vi "Take Your Seat.vi"(8 "error in (no error)":errorcluster, 10 "Front Panel Window:Panel Bounds":T1, 11 "Philosopher in":refnum<class "Philosopher.lvclass">) -> (0 "error out":errorcluster, 3 "Philosopher out":refnum<class "Philosopher.lvclass">)   [LabVIEW 2023, in "Philosopher.lvlib" / "Philosopher.lvclass"]
uses:
  Philosopher.lvclass
  <vilib>/Utility/miscctls.llb/LVRectTypeDef.ctl
  Philosopher.lvclass/Philosopher.ctl
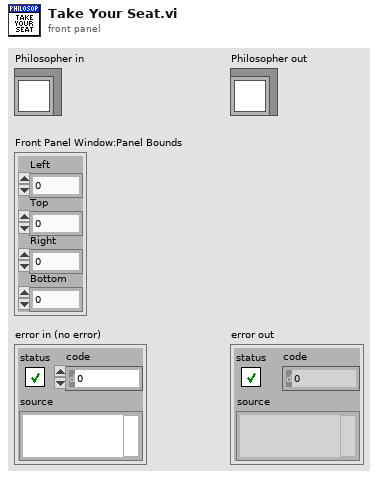
[diagram p1: front panel]
types:
  T1 = typedef "LVRectTypeDef.ctl" = cluster{"Left":i16, "Top":i16, "Right":i16, "Bottom":i16}
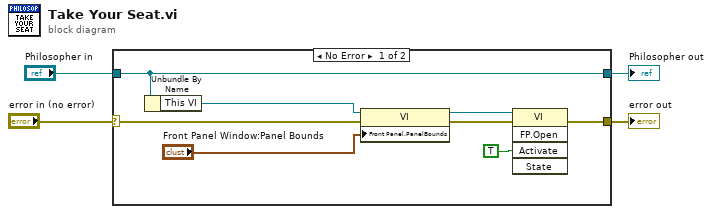
[diagram p0: block diagram]
diagram:
  n1 = case shown="No Error" "error in (no error)" {
    selector: "error in (no error)" -> [w12 w14]
    tunnel: [w5 w14] -> w3
    tunnel: [w11 w13] -> w1
    tunnel: "Philosopher in" -> [w11 w13]
    frame No Error {
      n2 = Unbundle By Name(w11) -> ("This VI"=w10:refnum<vi>)
      n3 = property class="VI"(reference=w10, error in=w12, "Front Panel.PanelBounds"="Front Panel Window:Panel Bounds") -> (reference out=w7:refnum<vi>, error out=w6:errorcluster)
      n4 = invoke on="Invoke Node" class="VI" method="FP.Open"(reference=w7, error in=w6, "Activate"=TRUE ("Activate?")) -> (error out=w5:errorcluster)  [unwired: 2 in, 4 out]
    }
    frame Error {
    }
  }
  "error out" <- w3
  "Philosopher out" <- w1
